vi "Servo_find_index.vi"(8 "error in (no error)":errorcluster, 9 "PWM":T1 items=["Invalid"=0, "PWM1"=1, "PWM2"=2, "PWM9"=9, "PWM10"=10]) -> (0 "error out":errorcluster, 1 "45 deg":dbl, 2 "0 deg":dbl, 3 "-45 deg":dbl)   [LabVIEW 2009, in "Servo.lvlib"]
uses:
  Servo.lvlib
  PWM/PWM_Name.ctl
  PWM.lvlib
panel:
  out "Output array":cluster{"value":dbl}[](array[cluster])
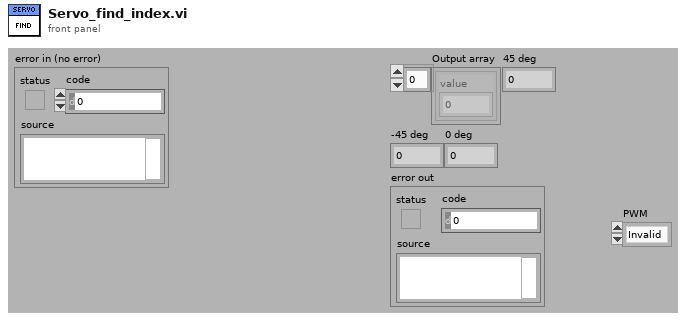
[diagram p1: front panel]
types:
  T1 = typedef "PWM.lvlib/PWM_Name.ctl" = u16
  T2 = cluster{"String":string, cluster{"value":dbl}[]}[]
  T3 = cluster{"[0]":cluster{"value":dbl}, "[1]":cluster{"value":dbl}, "[2]":cluster{"value":dbl}}
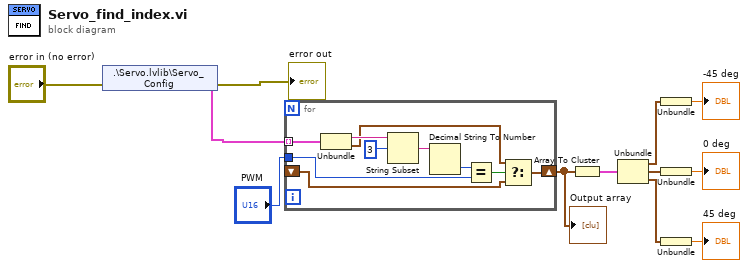
[diagram p0: block diagram]
diagram:
  n1 = shared-variable ".\\Servo.lvlib\\Servo_Config"(error in="error in (no error)") -> (w11:T2, error out=→"error out":errorcluster)
  n2 = for {
    tunnel: w11 -> [w22] mode=indexing
    tunnel: "PWM" -> [w18]
    shift-right: [w15] -> w10
    shift-left: _ -> [w14]
    n3 = Unbundle(w22) -> ("String"=w21:string, w17:cluster{"value":dbl}[])
    n4 = String Subset(string=w21, offset (0)=3) -> (substring=w19:string)  [unwired: 1 in]
    n5 = Decimal String To Number(string=w19) -> (number=w13:i32)  [unwired: 2 in, 1 out]
    n6 = Equal?(x=w13, y=w18) -> (x = y?=w16:bool)
    n7 = Select(t=w17, s=w16, f=w14) -> (s? t:f=w15:cluster{"value":dbl}[])
  }
  "Output array" <- w10
  n8 = Array To Cluster(array=w10) -> (cluster=w9:T3)
  n9 = Unbundle(w9) -> ("[0]"=w8:cluster{"value":dbl}, "[1]"=w7:cluster{"value":dbl}, "[2]"=w6:cluster{"value":dbl})
  n10 = Unbundle(w8) -> ("value"=→"-45 deg":dbl)
  n11 = Unbundle(w7) -> ("value"=→"0 deg":dbl)
  n12 = Unbundle(w6) -> ("value"=→"45 deg":dbl)
